vi "PRN Generation.vi"(8 "error in (no error)":errorcluster, 10 "PRN path":path, 11 "Cluster":T2) -> (0 "error out":errorcluster, 3 "PRN to Print":string)   [LabVIEW 2017]
uses:
  <vilib>/addons/database/Connection.llb/Conn ObjectReference.ctl
  <vilib>/addons/database/NI_Database_API.lvlib
panel:
  out "appended array":string[](array[string])
  out "concatenated string":string
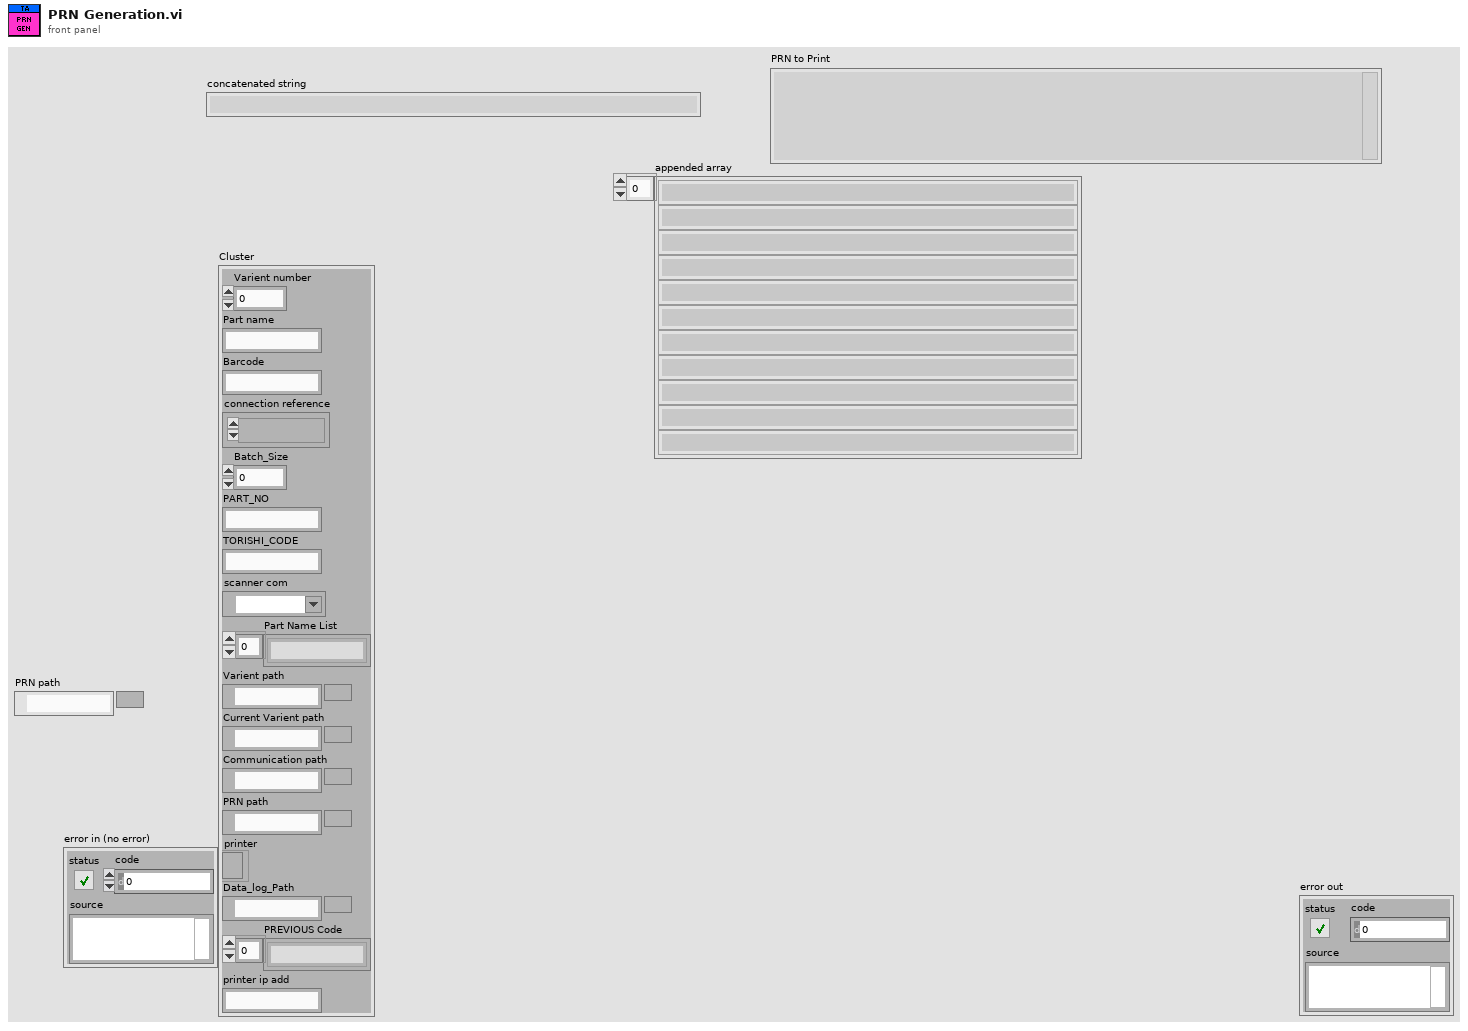
[diagram p1: front panel]
types:
  T1 = typedef "NI_Database_API.lvlib/Conn ObjectReference.ctl" = refnum<k1>
  T2 = cluster{"Varient number":u16, "Part name":string, "Barcode":string, "connection reference":T1, "Batch_Size":u16, "PART_NO":string, "TORISHI_CODE":string, "scanner com":refnum<visa-resource-name>, "Part Name List":string[], "Varient path":path, "Current Varient path":path, "Communication path":path, "PRN path":path, "printer":refnum<k5>, "Data_log_Path":path, "PREVIOUS Code":string[], "printer ip add":string}
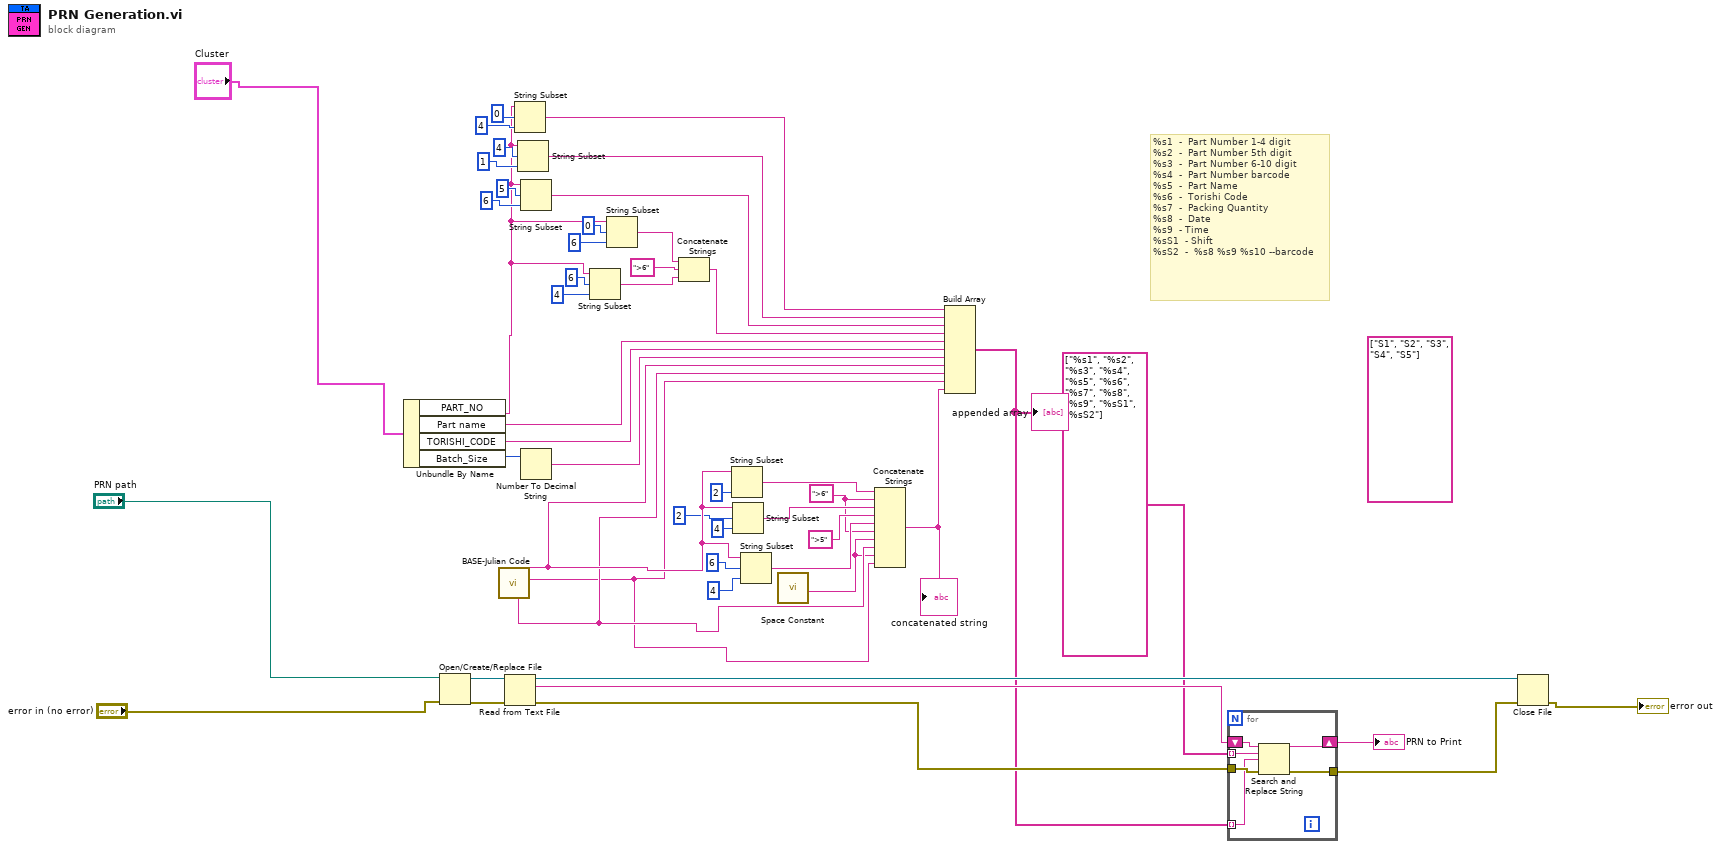
[diagram p0: block diagram]
diagram:
  w16 = ">6" ("string")
  (unwired) string[] ["S1", "S2", "S3", "S4", "S5"]
  # "%s1  -  Part Number 1-4 digit\n%s2  -  Part Number 5th digit\n%s3  -  Part Number 6-10 digit\n%s4  -  Part Number barcode\n%s5  -  Part Name\n%s6  -  Torishi Code\n%s7  -  Packing Quantity\n%s8  -  Date\n%s9  - Time\n%sS1  - Shift\n%sS2  -  %s8 %s9 %s10 --barcode"
  n1 = Unbundle By Name("Cluster") -> ("PART_NO"=w4:string, "Part name"=w29:string, "TORISHI_CODE"=w28:string, "Batch_Size"=w40:u16)
  n2 = Open/Create/Replace File(file path (use dialog)="PRN path", error in="error in (no error)") -> (refnum out=w47:refnum<file>, error out=w48:errorcluster)  [unwired: 4 in, 1 out]
  n3 = call "BASE-Julian Code.vi"() -> ("Shift"=w14:string, "Long time with :"=w15:string, "Long date with /"=w19:string)  [unwired: 6 in, 3 out]
  n4 = Read from Text File(file (use dialog)=w47, error in=w48) -> (refnum out=w49:refnum<file>, text=w45:string, error out=w43:errorcluster)  [unwired: 2 in, 1 out]
  n5 = String Subset(string=w4, offset (0)=0, length (rest)=4 ("length (rest)")) -> (substring=w32:string)
  n6 = String Subset(string=w4, offset (0)=4, length (rest)=1 ("length (rest)")) -> (substring=w31:string)
  n7 = String Subset(string=w4, offset (0)=5, length (rest)=6 ("length (rest)")) -> (substring=w30:string)
  n8 = Number To Decimal String(number=w40) -> (decimal integer string=w27:string)  [unwired: 1 in]
  n9 = String Subset(string=w4, offset (0)=6, length (rest)=4 ("length (rest)")) -> (substring=w5:string)
  n10 = String Subset(string=w4, offset (0)=0, length (rest)=6 ("length (rest)")) -> (substring=w9:string)
  n11 = Concatenate Strings(w9, ">6" ("string"), w5) -> (w3:string)
  n12 = String Subset(string=w19, length (rest)=2 ("length (rest)")) -> (substring=w25:string)  [unwired: 1 in]
  n13 = String Subset(string=w19, offset (0)=2, length (rest)=4 ("length (rest)")) -> (substring=w22:string)
  n14 = String Subset(string=w19, offset (0)=6, length (rest)=4 ("length (rest)")) -> (substring=w17:string)
  n15 = call <vilib>:"Space Constant.vi"() -> ("String"=w2:string)
  n16 = Concatenate Strings(w25, w16, w22, ">5" ("string"), w17, w16, w2, w15, w2, w14) -> (w13:string)
  "concatenated string" <- w13
  n17 = Build Array(w32, w31, w30, w3, w29, w28, w27, w19, w15, w14, w13) -> (w26:string[])
  "appended array" <- w26
  n18 = for {
    shift-right: [w55] -> w44
    shift-left: w45 -> [w56]
    tunnel: w43 -> [w54]
    tunnel: [w53] -> w42
    tunnel: string[] ["%s1", "%s2", "%s3", "%s4", "%s5", "%s6", "%s7", "%s8", "%s9", "%sS1", "%sS2"] -> [w52] mode=indexing
    tunnel: w26 -> [w51] mode=indexing
    n19 = Search and Replace String(input string=w56, search string=w52, replace string=w51, error in=w54) -> (result string=w55:string, error out=w53:errorcluster)  [unwired: 4 in, 2 out]
  }
  "PRN to Print" <- w44
  n20 = Close File(refnum=w49, error in=w42) -> (error out=→"error out":errorcluster)  [unwired: 1 out]
